vi "Verileri GUI'ye Gönder_Flicker.vi"(3 "Uygulanan Deðerler":dbl[][](array[numeric])=[[0.0, 0.0, 0.0, 0.0], [0.0, 0.0, 0.0, 0.0]], 4 "FD2 C":dbl, 5 "FD2 B":dbl, 6 "FD2 A":dbl, 7 "FD1 C":dbl, 8 "FD1 B":dbl, 9 "FD1 A":dbl, 10 "Limit Deger":dbl, 11 "Ölçüm No":u16) -> ()   [LabVIEW 2014]
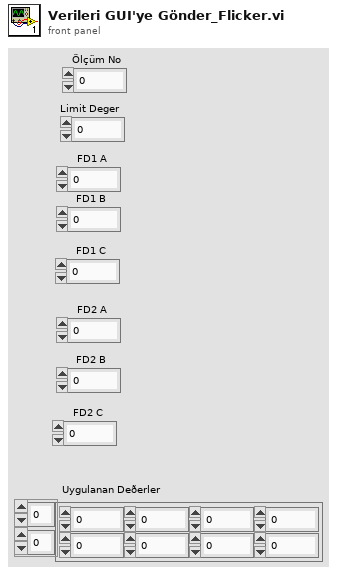
[diagram p1: front panel]
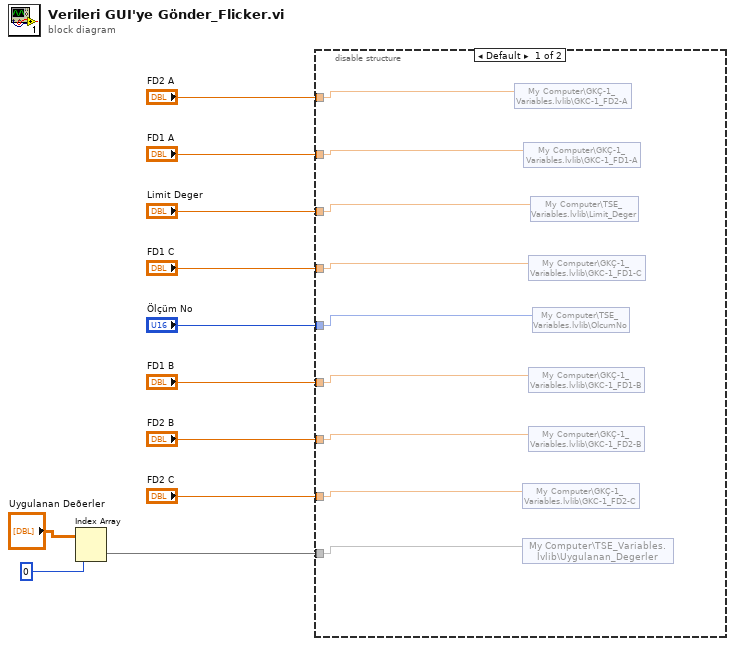
[diagram p0: block diagram]
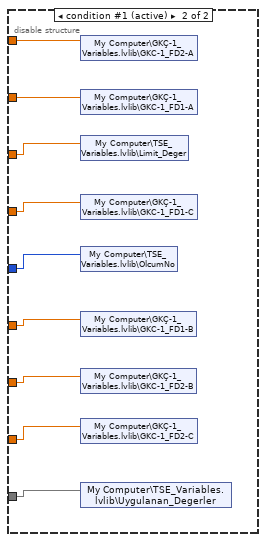
[diagram p2: hidden frame]
diagram:
  n1 = Index Array(array="Uygulanan Deðerler", index (row)=0) -> (element=w1:dbl[])  [unwired: 1 in]
  n2 = disable-structure shown="Default" {
    disable-tunnel: "FD1 C" -> [w17 w26]
    disable-tunnel: "Limit Deger" -> [w18 w27]
    disable-tunnel: "FD2 A" -> [w20 w29]
    disable-tunnel: "FD1 A" -> [w19 w28]
    disable-tunnel: "Ölçüm No" -> [w16 w25]
    disable-tunnel: "FD1 B" -> [w15 w24]
    disable-tunnel: "FD2 B" -> [w14 w23]
    disable-tunnel: "FD2 C" -> [w13 w22]
    disable-tunnel: w1 -> [w12 w21]
    frame condition #0 {
      n3 = shared-variable "My Computer\\GKÇ-1_Variables.lvlib\\GKC-1_FD2-A"(w20) -> ()  [unwired: 1 in, 1 out]
      n4 = shared-variable "My Computer\\GKÇ-1_Variables.lvlib\\GKC-1_FD2-C"(w13) -> ()  [unwired: 1 in, 1 out]
      n5 = shared-variable "My Computer\\TSE_Variables.lvlib\\Uygulanan_Degerler"(w12) -> ()  [unwired: 1 in, 1 out]
      n6 = shared-variable "My Computer\\GKÇ-1_Variables.lvlib\\GKC-1_FD1-A"(w19) -> ()  [unwired: 1 in, 1 out]
      n7 = shared-variable "My Computer\\GKÇ-1_Variables.lvlib\\GKC-1_FD1-C"(w17) -> ()  [unwired: 1 in, 1 out]
      n8 = shared-variable "My Computer\\GKÇ-1_Variables.lvlib\\GKC-1_FD1-B"(w15) -> ()  [unwired: 1 in, 1 out]
      n9 = shared-variable "My Computer\\GKÇ-1_Variables.lvlib\\GKC-1_FD2-B"(w14) -> ()  [unwired: 1 in, 1 out]
      n10 = shared-variable "My Computer\\TSE_Variables.lvlib\\Limit_Deger"(w18) -> ()  [unwired: 1 in, 1 out]
      n11 = shared-variable "My Computer\\TSE_Variables.lvlib\\OlcumNo"(w16) -> ()  [unwired: 1 in, 1 out]
    }
    frame condition #1 (active) {
      n12 = shared-variable "My Computer\\GKÇ-1_Variables.lvlib\\GKC-1_FD2-A"(w29) -> ()  [unwired: 1 in, 1 out]
      n13 = shared-variable "My Computer\\GKÇ-1_Variables.lvlib\\GKC-1_FD1-A"(w28) -> ()  [unwired: 1 in, 1 out]
      n14 = shared-variable "My Computer\\TSE_Variables.lvlib\\Limit_Deger"(w27) -> ()  [unwired: 1 in, 1 out]
      n15 = shared-variable "My Computer\\GKÇ-1_Variables.lvlib\\GKC-1_FD1-C"(w26) -> ()  [unwired: 1 in, 1 out]
      n16 = shared-variable "My Computer\\TSE_Variables.lvlib\\OlcumNo"(w25) -> ()  [unwired: 1 in, 1 out]
      n17 = shared-variable "My Computer\\GKÇ-1_Variables.lvlib\\GKC-1_FD1-B"(w24) -> ()  [unwired: 1 in, 1 out]
      n18 = shared-variable "My Computer\\GKÇ-1_Variables.lvlib\\GKC-1_FD2-B"(w23) -> ()  [unwired: 1 in, 1 out]
      n19 = shared-variable "My Computer\\GKÇ-1_Variables.lvlib\\GKC-1_FD2-C"(w22) -> ()  [unwired: 1 in, 1 out]
      n20 = shared-variable "My Computer\\TSE_Variables.lvlib\\Uygulanan_Degerler"(w21) -> ()  [unwired: 1 in, 1 out]
    }
  }
